vi "1mhztimingsource_1000dt.vi"() -> (0 "max jitter (uS)":dbl format="%.2f", 1 "mean time (uS)":dbl format="%.2f", 2 "standard deviation (uS)":dbl format="%.2f", 3 "execution histogram":T1(graph), 4 "Error":errorcluster, 5 "execution times (uS)":dbl[](graph))   [LabVIEW 2013]
uses:
  <vilib>/platform/TimedLoop/XDataNode/XDataNode.xnode
  <vilib>/Platform/TimedLoop/XDataNode/nitl_modes.ctl
  <vilib>/Platform/TimedLoop/XDataNode/XDNodeRunTimeDep.lvlib
  <vilib>/Platform/TimedLoop/XDataNode/wakeup.ctl
  <vilib>/Platform/TimedLoop/XDataNode/timing_clust.ctl
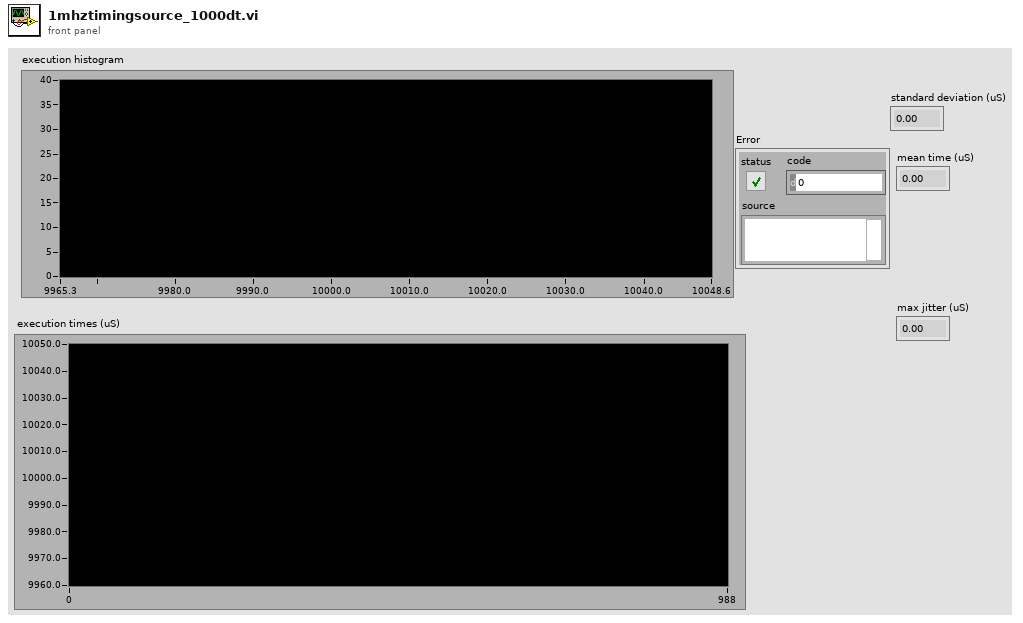
[diagram p1: front panel]
types:
  T1 = cluster{"X Values":dbl[], "Histogram: h(x)":i32[]}
  T2 = typedef "XDNodeRunTimeDep.lvlib/timing_clust.ctl" = cluster{"Expected End [f-1]":u64, "Actual End [f-1]":u64, "Finished Late? [f-1]":bool, "Expected End [i-1]":u64, "Actual End [i-1]":u64, "Finished Late? [i-1]":bool, "Expected Start [i]":u64, "Actual Start [i]":u64, "Expected Start [f]":u64, "Actual Start [f]":u64, "Source Name":string, "Structure Name":string, "Period":i64, "Deadline":i64, "Offset":i64, "Start":i64, "Priority":i32, "Timeout":i32, "Mode":T3, "Wakeup Reason":T4, "Error":errorcluster, "Source Type":string, "Secondary Source Type":string, "Global End Time":u64, "Global Start Time":u64, "Frame Duration":u64, "Iteration Duration":u64, "Assigned CPU":i32, "I/O Scan Engine Mode":u32}
  T3 = typedef "XDNodeRunTimeDep.lvlib/nitl_modes.ctl" = enum32{"No Change", "Process missed periods, maintain original phase", "Discard missed periods, maintain original phase", "Process missed periods, ignore original phase", "Discard missed periods, ignore original phase"}
  T4 = typedef "XDNodeRunTimeDep.lvlib/wakeup.ctl" = enum32{"Normal", "Aborted", "Asynchronous wakeup", "Timing source error", "Timed loop error", "Timeout"}
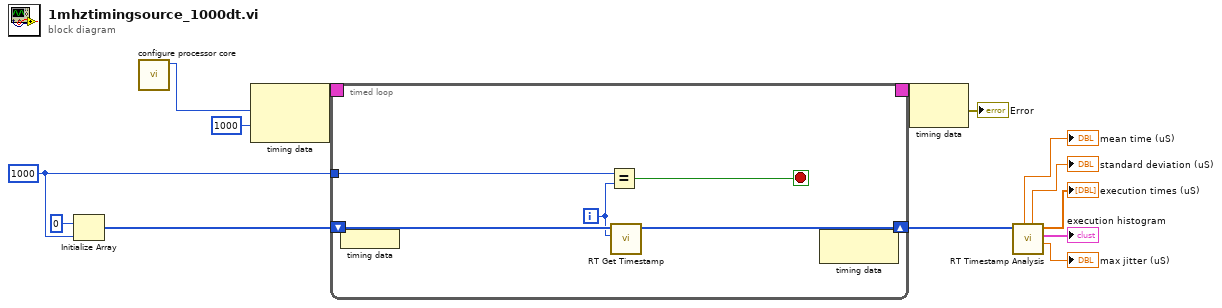
[diagram p0: block diagram]
diagram:
  w12 = 1000 ("x")
  n1 = Initialize Array(u64 0, w12) -> (w13:u64[])
  n2 = call "configure processor core.vi"() -> ("Processor"=w2:i32)  [unwired: 11 in]
  n3 = node-c288(w2, i64 1000 ("Period")) -> (w5:T2)
  n4 = timed-loop {
    timing: w5 -> [_]
    timing-out: [_] -> w4
    shift-right: [w16] -> w11
    shift-left: w13 -> [w17]
    tunnel: w12 -> [w19]
    i -> [w15]
    stop <- w18 stop-if-true
    n5 = node-c288() -> ()  [unwired: 1 in]
    n6 = Equal?(x=w19, y=w15) -> (x = y?=w18:bool)
    n7 = call <vilib>:"RT Get Timestamp.vi"("iteration"=w15, "timestamp array in"=w17) -> ("timestamp array out"=w16:u64[])  [unwired: 8 in, 1 out]
    n8 = node-c288() -> ()  [unwired: 1 in, 1 out]
  }
  n9 = node-c288(w4) -> (→"Error":errorcluster)
  n10 = call <vilib>:"RT Timestamp Analysis.vi"("timestamp array"=w11) -> ("max jitter (uS)"=→"max jitter (uS)":dbl, "execution histogram"=→"execution histogram":T1, "execution times (uS)"=→"execution times (uS)":dbl[], "standard deviation (uS)"=→"standard deviation (uS)":dbl, "mean time (uS)"=→"mean time (uS)":dbl)  [unwired: 5 in, 1 out]
